vi "Query_System_Folder_Path.vi"(8 "error in (no error)":errorcluster, 10 "nFolder":u8, 11 "Dest_NI_MSIPath in":refnum<class "Dest_NI_MSIPath.lvclass">) -> (0 "error out":errorcluster, 2 "path":path, 3 "Dest_NI_MSIPath out":refnum<class "Dest_NI_MSIPath.lvclass">)   [LabVIEW 2020, in "Dest_NI_MSIPath.lvclass"]
uses:
  <vilib>/AppBuilder/IB_Classes/Dest_NI_MSIPath/Dest_NI_MSIPath.lvclass
  <vilib>/AppBuilder/IB_Classes/Dest_NI_MSIPath/Dest_NI_MSIPath.lvclass/Dest_NI_MSIPath.ctl
  shfolder.dll
  <vilib>/AppBuilder/IB_Classes/Destination/niLabel/niLabel.lvclass
  e:/builds/penguin/labview/branches/2020/dev/dist/vi.lib/AppBuilder/IB_Classes/Destination/niLabel/niLabel.lvclass
  e:/builds/penguin/labview/branches/2020/dev/dist/vi.lib/AppBuilder/IB_Classes/Destination/IB_Destination.lvclass
  e:/builds/penguin/labview/branches/2020/dev/dist/vi.lib/AppBuilder/IB_Classes/Dest_NI_MSIPath/Dest_NI_MSIPath.lvclass
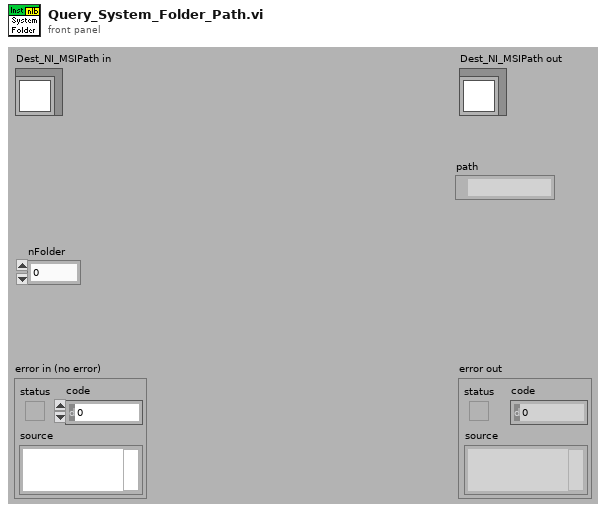
[diagram p1: front panel]
types:
  T1 = typedef "IB_Dest_niLabel.ctl" = cluster{"local path":path}
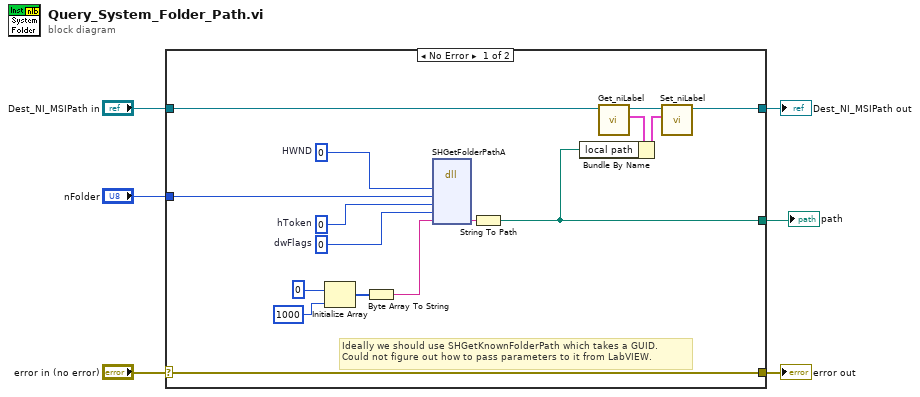
[diagram p0: block diagram]
diagram:
  n1 = case shown="No Error" "error in (no error)" {
    selector: "error in (no error)" -> [w22 w24]
    tunnel: [w22 w24] -> w5
    tunnel: [w11 w23] -> w3
    tunnel: "Dest_NI_MSIPath in" -> [w10 w23]
    tunnel: "nFolder" -> [w13 _]
    tunnel: [w12 _] -> w1
    frame No Error {
      w19 = 0  # dwFlags
      w20 = 0  # hToken
      w14 = 0  # HWND
      # "Ideally we should use SHGetKnownFolderPath which takes a GUID.\nCould not figure out how to pass parameters to it from LabVIEW."
      n2 = Initialize Array(u8 0, 1000 ("dimension size")) -> (w16:u8[])
      n3 = Byte Array To String(unsigned byte array=w16) -> (string=w15:string)
      n4 = dll-call lib="shfolder.dll" fn="SHGetFolderPathA"("HWND"=w14, "nFolder"=w13, "hToken"=w20, "dwFlags"=w19, "pszPath"=w15) -> ("pszPath"=w21:string)  [unwired: 8 in, 2 out]
      n5 = String To Path(string=w21) -> (path=w12:path)
      n6 = call <vilib>:"Get_niLabel.vi"("niLabel in"=w10) -> ("data"=w9:T1, "niLabel out"=w7:refnum<class "Dest_NI_MSIPath.lvclass">)  [unwired: 8 in, 1 out]
      n7 = Bundle By Name(cluster=w9, "local path"=w12) -> (w8:T1)
      n8 = call <vilib>:"Set_niLabel.vi"("data"=w8, "niLabel in"=w7) -> ("niLabel out"=w11:refnum<class "Dest_NI_MSIPath.lvclass">)  [unwired: 8 in, 1 out]
    }
    frame Error {
    }
  }
  "error out" <- w5
  "Dest_NI_MSIPath out" <- w3
  "path" <- w1
